vi "Airmar WS.vi"(8 "error in":errorcluster) -> (0 "error out":errorcluster)   [LabVIEW 2015]
uses:
  Devices/Airmar/Airmar WS.lvclass
  Reusable/Session Log/System Log.lvclass
  Devices/Airmar/Data/Airmar Data.lvclass
  <userlib>/_Session Fwk/Session - Root.lvclass
  Reusable/Session APIs/Serial/Serial Session.lvclass
  Reusable/Session APIs/File Access/Config Data/Config Data.lvclass
  Reusable/Session APIs/File Access/Config Data/Config Session.ctl
  <vilib>/Platform/TimedLoop/XDataNode/XDataNode.xnode
  <vilib>/Platform/TimedLoop/XDataNode/nitl_modes.ctl
  <vilib>/Platform/TimedLoop/XDataNode/XDNodeRunTimeDep.lvlib
  <vilib>/Platform/TimedLoop/XDataNode/wakeup.ctl
  <vilib>/Platform/TimedLoop/XDataNode/timing_clust.ctl
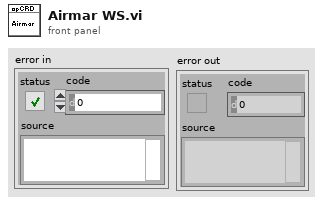
[diagram p1: front panel]
types:
  T1 = typedef "Config Data.lvclass/Config Session.ctl" = refnum<data-value>
  T2 = typedef "Session - Root.lvclass/Session Handle.ctl" = refnum<data-value>
  T3 = typedef "XDNodeRunTimeDep.lvlib/timing_clust.ctl" = cluster{"Expected End [f-1]":u64, "Actual End [f-1]":u64, "Finished Late? [f-1]":bool, "Expected End [i-1]":u64, "Actual End [i-1]":u64, "Finished Late? [i-1]":bool, "Expected Start [i]":u64, "Actual Start [i]":u64, "Expected Start [f]":u64, "Actual Start [f]":u64, "Source Name":string, "Structure Name":string, "Period":i64, "Deadline":i64, "Offset":i64, "Start":i64, "Priority":i32, "Timeout":i32, "Mode":T4, "Wakeup Reason":T5, "Error":errorcluster, "Source Type":string, "Secondary Source Type":string, "Global End Time":u64, "Global Start Time":u64, "Frame Duration":u64, "Iteration Duration":u64, "Assigned CPU":i32, "I/O Scan Engine Mode":u32}
  T4 = typedef "XDNodeRunTimeDep.lvlib/nitl_modes.ctl" = enum32{"No Change", "Process missed periods, maintain original phase", "Discard missed periods, maintain original phase", "Process missed periods, ignore original phase", "Discard missed periods, ignore original phase"}
  T5 = typedef "XDNodeRunTimeDep.lvlib/wakeup.ctl" = enum32{"Normal", "Aborted", "Asynchronous wakeup", "Timing source error", "Timed loop error", "Timeout"}
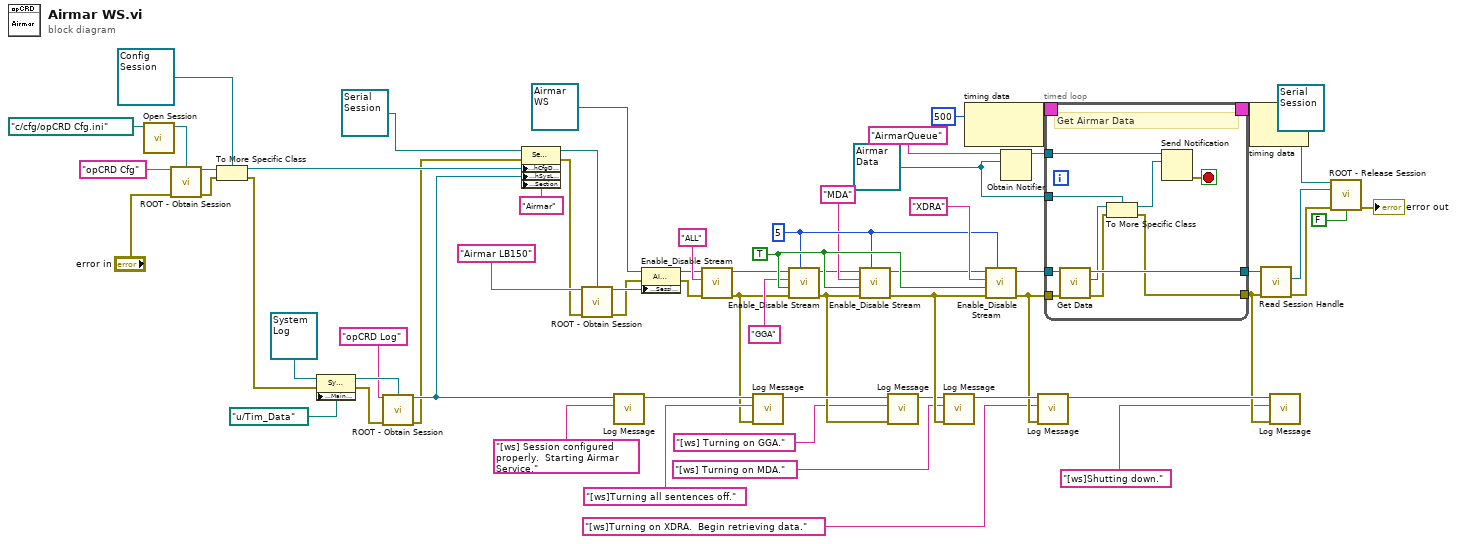
[diagram p0: block diagram]
diagram:
  w4 = refnum<class "Airmar Data.lvclass"> refnum ("Airmar Data")
  w61 = i16 5 ("time")
  w62 = TRUE ("Enable?")
  n1 = call "Open Session.vi"("Path"=path "c:/cfg/opCRD Cfg.ini") -> ("Config Data"=w11:refnum<class "Config Data.lvclass">)  [unwired: 9 in, 1 out]
  n2 = call <userlib>:"ROOT - Obtain Session.vi"("Session Name ()"="opCRD Cfg", "OBJ - Session"=w11, "error in (no error)"="error in") -> ("Session Handle"=w14:T2, "error out"=w15:errorcluster)  [unwired: 10 in, 1 out]
  n3 = To More Specific Class(target class=T1 refnum ("Session Handle"), reference=w14, error in=w15) -> (specific class reference=w10:T1, error out=w7:errorcluster)
  n4 = property class="Sys Log"(reference=refnum<class "System Log.lvclass"> refnum ("Sys Log"), error in=w7, "Accessors:Main Path"=path "u:/Tim_Data" ("RD Data Path")) -> (reference out=w32:refnum<class "System Log.lvclass">, error out=w31:errorcluster)
  n5 = call <userlib>:"ROOT - Obtain Session.vi"("Session Name ()"="opCRD Log", "OBJ - Session"=w32, "error in (no error)"=w31) -> ("Session Handle"=w21:T2, "error out"=w6:errorcluster)  [unwired: 10 in, 1 out]
  n6 = property class="Serial Session"(reference=refnum<class "Serial Session.lvclass"> refnum ("Serial Session in"), error in=w6, "Accessors:hCfgData"=w10, "Accessors:hSysLog"=w21, "Accessors:Section"="Airmar" ("Section")) -> (reference out=w19:refnum<class "Serial Session.lvclass">, error out=w9:errorcluster)
  n7 = call <userlib>:"ROOT - Obtain Session.vi"("Session Name ()"="Airmar LB150", "OBJ - Session"=w19, "error in (no error)"=w9) -> ("Session Handle"=w18:T2, "error out"=w5:errorcluster)  [unwired: 10 in, 1 out]
  n8 = call "Log Message.vi"("MSG In"="[ws] Session configured properly.  Starting Airmar Service.", "session in"=w21) -> ("session out"=w51:T2)  [unwired: 8 in, 1 out]
  n9 = property class="Airmar WS"(reference=refnum<class "Airmar WS.lvclass"> refnum ("Airmar WS in"), error in=w5, "Accessors:Session Handle"=w18) -> (reference out=w53:refnum<class "Airmar WS.lvclass">, error out=w29:errorcluster)
  n10 = call "Enable_Disable Stream.vi"("error in"=w29, "String"="ALL", "Airmar WS in"=w53) -> ("error out"=w49:errorcluster, "Airmar WS out"=w55:refnum<class "Airmar WS.lvclass">)  [unwired: 7 in]
  n11 = call "Log Message.vi"("error in"=w49, "MSG In"="[ws]Turning all sentences off.", "session in"=w51) -> ("session out"=w48:T2)  [unwired: 7 in, 1 out]
  n12 = call "Enable_Disable Stream.vi"("time"=w61, "error in"=w49, "Enable?"=w62, "String"="GGA", "Airmar WS in"=w55) -> ("error out"=w47:errorcluster, "Airmar WS out"=w57:refnum<class "Airmar WS.lvclass">)  [unwired: 5 in]
  n13 = call "Enable_Disable Stream.vi"("time"=w61, "error in"=w47, "Enable?"=w62, "String"="MDA", "Airmar WS in"=w57) -> ("error out"=w45:errorcluster, "Airmar WS out"=w60:refnum<class "Airmar WS.lvclass">)  [unwired: 5 in]
  n14 = call "Log Message.vi"("error in"=w47, "MSG In"="[ws] Turning on GGA.", "session in"=w48) -> ("session out"=w44:T2)  [unwired: 7 in, 1 out]
  n15 = call "Log Message.vi"("error in"=w45, "MSG In"="[ws] Turning on MDA.", "session in"=w44) -> ("session out"=w42:T2)  [unwired: 7 in, 1 out]
  n16 = node-c288(i64 500 ("Period")) -> (w3:T3)
  n17 = call "Enable_Disable Stream.vi"("time"=w61, "error in"=w45, "Enable?"=w62, "String"="XDRA", "Airmar WS in"=w60) -> ("error out"=w41:errorcluster, "Airmar WS out"=w64:refnum<class "Airmar WS.lvclass">)  [unwired: 5 in]
  n18 = Obtain Notifier(name (unnamed)="AirmarQueue", notification data type=w4) -> (notifier out=w35:refnum<notifier>)  [unwired: 2 in, 2 out]
  n19 = call "Log Message.vi"("error in"=w41, "MSG In"="[ws]Turning on XDRA.  Begin retrieving data.", "session in"=w42) -> ("session out"=w39:T2)  [unwired: 7 in, 1 out]
  n20 = timed-loop {
    tunnel: w64 -> [w74]
    tunnel: w35 -> [w73]
    tunnel: [w71] -> w59
    tunnel: w41 -> [w70]
    tunnel: [w65] -> w38
    tunnel: w4 -> [w68]
    timing: w3 -> [_]
    timing-out: [_] -> w2
    stop <- w72 stop-if-true
    # "Get Airmar Data"
    n21 = call-dynamic "Get Data.vi"("error in"=w70, "Airmar WS in"=w74) -> ("error out"=w66:errorcluster, "Data"=w69:refnum<class "Data.lvclass">, "Airmar WS out"=w71:refnum<class "Airmar WS.lvclass">)  [unwired: 7 in]
    n22 = To More Specific Class(target class=w68, reference=w69, error in=w66) -> (specific class reference=w67:refnum<class "Airmar Data.lvclass">, error out=w65:errorcluster)
    n23 = Send Notification(notification=w67, notifier=w73) -> (error out=w72:errorcluster)  [unwired: 1 in, 1 out]
  }
  n24 = node-c288(w2) -> ()  [unwired: 1 out]
  n25 = call "Read Session Handle.vi"("error in (no error)"=w38, "Airmar WS in"=w59) -> ("error out"=w25:errorcluster, "hSerial"=w28:T2)  [unwired: 7 in, 1 out]
  n26 = call "Log Message.vi"("error in"=w38, "MSG In"="[ws]Shutting down.", "session in"=w39) -> ()  [unwired: 7 in, 2 out]
  n27 = call <userlib>:"ROOT - Release Session.vi"("OBJ - Session in"=refnum<class "Serial Session.lvclass"> refnum ("Serial Session"), "Session Handle in"=w28, "error in (no error)"=w25, "force destroy? (F)"=FALSE) -> ("error out"=→"error out":errorcluster)  [unwired: 10 in, 1 out]
